vi "String.2D to CSV ready 2D.vi"(11 "2D In":string[][](array[string])) -> (3 "2D In Out":string[][](array[string]))   [LabVIEW 2018]
uses:
  <vilib>/KATE/Files/File Utils.lvlib
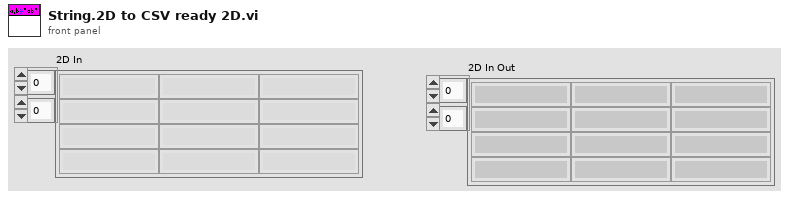
[diagram p1: front panel]
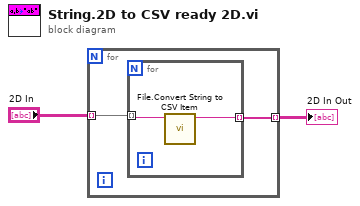
[diagram p0: block diagram]
diagram:
  n1 = for {
    tunnel: "2D In" -> [w4] mode=indexing
    tunnel: [w3] -> w1 mode=indexing
    n2 = for {
      tunnel: w4 -> [w6] mode=indexing
      tunnel: [w5] -> w3 mode=indexing
      n3 = call <vilib>:"File.Convert String to CSV Item.vi"("String"=w6) -> ("String Out"=w5:string)  [unwired: 10 in]
    }
  }
  "2D In Out" <- w1
